vi "PowerSupplyVoltageControl.vi"(11 "Manual Range(0.00)":dbl format="%.2f") -> (0 "error out":errorcluster)   [LabVIEW 2009]
uses:
  <instrlib>/BK Precision 91xx Series/BK Precision 91xx Series.lvlib
panel:
  in  "Reset (True)":bool=TRUE
  in  "Unit(V)":u16(ring) items=["V", "mV", "kV", "A", "mA"]
  in  "Enable Output (T: Enable)":bool=TRUE
  in  "Function(0:Voltage)":u16(ring) items=["Voltage", "Current"]
  in  "ID Query (True)":bool=TRUE
  in  "VISA resource name":refnum<visa-resource-name>
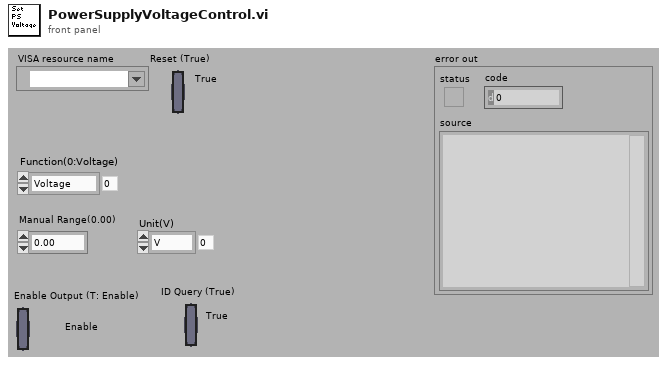
[diagram p1: front panel]
types:
  T1 = cluster{"Parity(0:none)":u16, "Baud Rate (9600)":u16, "Data Bits(8)":u16, "Flow Control(None)":u16, " Stop Bits(1.0)":u16}
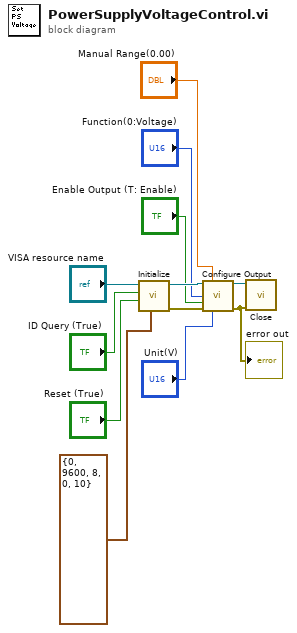
[diagram p0: block diagram]
diagram:
  n1 = call <instrlib>:"Initialize.vi"("Serial Configuration"=T1 {"Parity(0:none)"=0, "Baud Rate (9600)"=9600, "Data Bits(8)"=8, "Flow Control(None)"=0, " Stop Bits(1.0)"=10}, "Reset (True)"="Reset (True)", "ID Query (True)"="ID Query (True)", "VISA resource name"="VISA resource name") -> ("error out"=w9:errorcluster, "VISA resource name out"=w12:refnum<visa-resource-name>)  [unwired: 6 in]
  n2 = call <instrlib>:"Configure Output.vi"("VISA resource name"=w12, "Manual Range(0.00)"="Manual Range(0.00)", "Function(0:Voltage)"="Function(0:Voltage)", "Enable Output (T: Enable)"="Enable Output (T: Enable)", "error in (no error)"=w9, "Unit(V)"="Unit(V)") -> ("VISA resource name out"=w11:refnum<visa-resource-name>, "error out"=w10:errorcluster)  [unwired: 8 in]
  "error out" <- w10
  n3 = call <instrlib>:"Close.vi"("error in (no error)"=w10, "VISA resource name"=w11) -> ()  [unwired: 9 in, 1 out]
